vi "Session&Bearer_operation.vi"(10 "NewVal":T1(array[cluster]), 11 "OldVal":T1(array[cluster])) -> (1 "output array":T1(array[cluster]), 2 "Bearer":i32, 3 "Delete Index":i32)   [LabVIEW 2021]
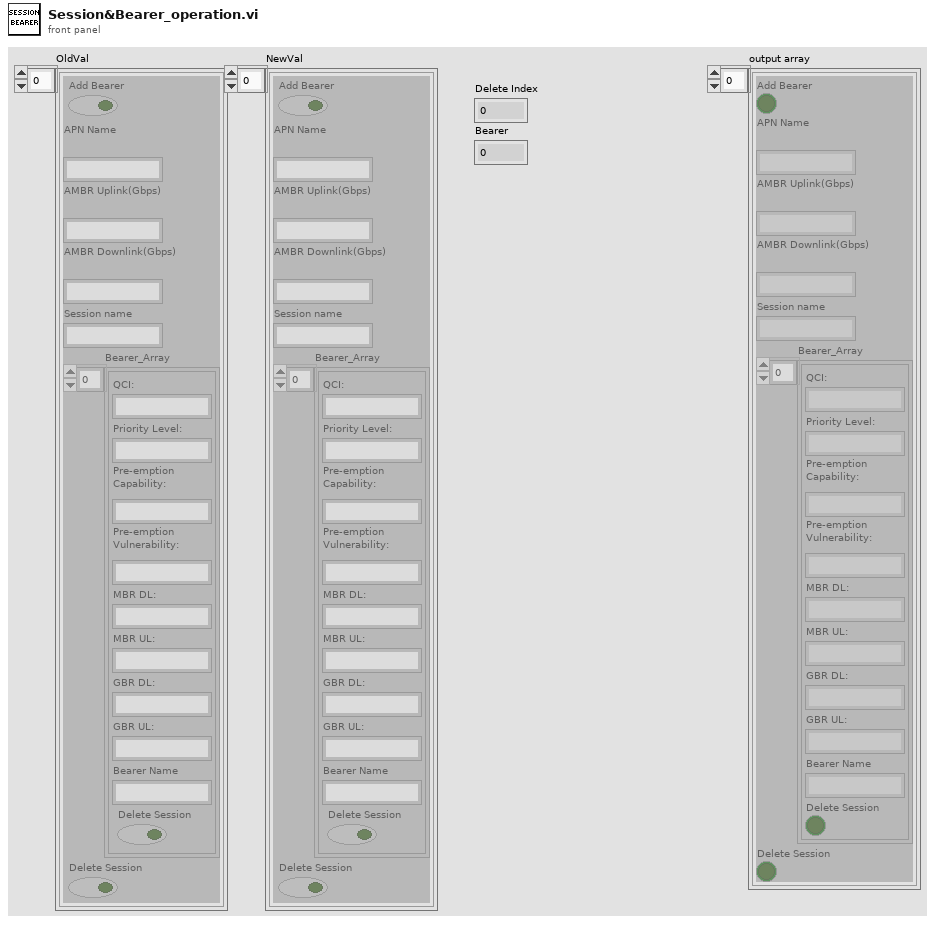
[diagram p1: front panel]
types:
  T1 = cluster{"Add Bearer":bool, "APN Name\n":string, "AMBR Uplink(Gbps)\n":string, "AMBR Downlink(Gbps)\n":string, "Session name":string, "Bearer_Array":cluster{"QCI:":string, "Priority Level:":string, "Pre-emption\nCapability:":string, "Pre-emption\nVulnerability:":string, "MBR DL:":string, "MBR UL:":string, "GBR DL:":string, "GBR UL:":string, "Bearer Name":string, "Delete Session":bool}[], "Delete Session":bool}[]
  T2 = cluster{"Add Bearer":bool, "APN Name\n":string, "AMBR Uplink(Gbps)\n":string, "AMBR Downlink(Gbps)\n":string, "Session name":string, "Bearer_Array":cluster{"QCI:":string, "Priority Level:":string, "Pre-emption\nCapability:":string, "Pre-emption\nVulnerability:":string, "MBR DL:":string, "MBR UL:":string, "GBR DL:":string, "GBR UL:":string, "Bearer Name":string, "Delete Session":bool}[], "Delete Session":bool}
  T3 = cluster{"QCI:":string, "Priority Level:":string, "Pre-emption\nCapability:":string, "Pre-emption\nVulnerability:":string, "MBR DL:":string, "MBR UL:":string, "GBR DL:":string, "GBR UL:":string, "Bearer Name":string, "Delete Session":bool}[]
  T4 = cluster{"QCI:":string, "Priority Level:":string, "Pre-emption\nCapability:":string, "Pre-emption\nVulnerability:":string, "MBR DL:":string, "MBR UL:":string, "GBR DL:":string, "GBR UL:":string, "Bearer Name":string, "Delete Session":bool}
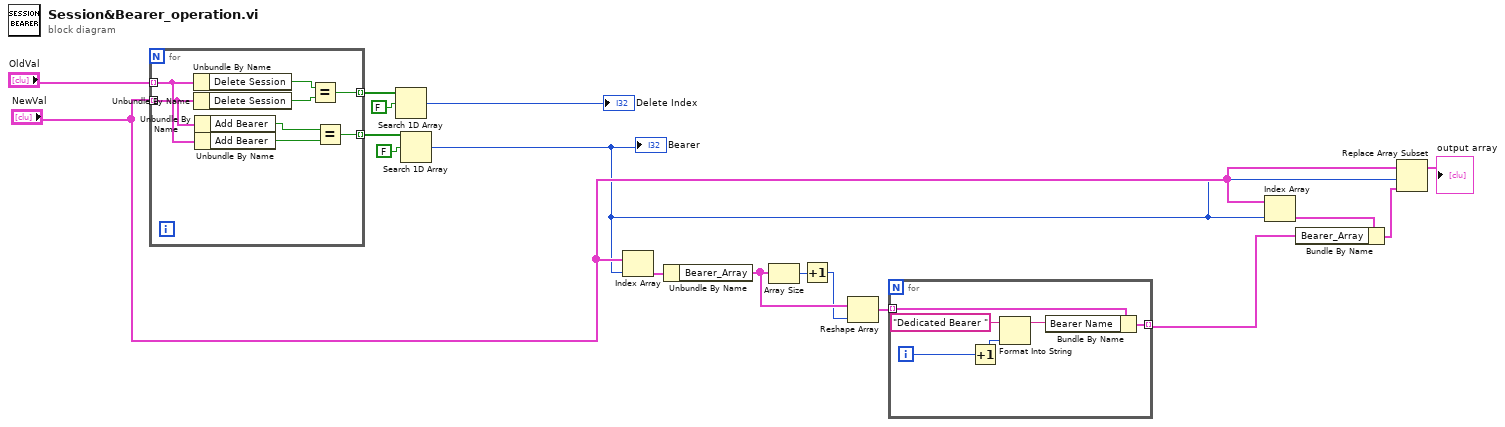
[diagram p0: block diagram]
diagram:
  n1 = for {
    tunnel: "OldVal" -> [w19] mode=indexing
    tunnel: "NewVal" -> [w18] mode=indexing
    tunnel: [w23] -> w17 mode=indexing
    tunnel: [w20] -> w13 mode=indexing
    n2 = Unbundle By Name(w19) -> ("Delete Session"=w25:bool)
    n3 = Unbundle By Name(w18) -> ("Delete Session"=w24:bool)
    n4 = Unbundle By Name(w18) -> ("Add Bearer"=w22:bool)
    n5 = Unbundle By Name(w19) -> ("Add Bearer"=w21:bool)
    n6 = Equal?(x=w25, y=w24) -> (x = y?=w23:bool)
    n7 = Equal?(x=w22, y=w21) -> (x = y?=w20:bool)
  }
  n8 = Search 1D Array(1D array=w17, element=FALSE ("x = y?")) -> (index of element=→"Delete Index":i32)  [unwired: 1 in]
  n9 = Search 1D Array(1D array=w13, element=FALSE ("x = y?")) -> (index of element=w1:i32)  [unwired: 1 in]
  "Bearer" <- w1
  n10 = Index Array(array="NewVal", index=w1) -> (element=w12:T2)
  n11 = Unbundle By Name(w12) -> ("Bearer_Array"=w11:T3)
  n12 = Array Size(array=w11) -> (size(s)=w10:i32)
  n13 = Increment(x=w10) -> (x+1=w9:i32)
  n14 = Reshape Array(w11, w9) -> (w8:T3)
  n15 = for {
    tunnel: w8 -> [w31] mode=indexing
    tunnel: [w26] -> w4 mode=indexing
    i -> [w28]
    n16 = Increment(x=w28) -> (x+1=w27:i32)
    n17 = Format Into String(initial string="Dedicated Bearer ", w27) -> (resulting string=w30:string)  [unwired: 2 in, 1 out]
    n18 = Bundle By Name(cluster=w31, "Bearer Name"=w30) -> (w26:T4)
  }
  n19 = Index Array(array="NewVal", index=w1) -> (element=w5:T2)
  n20 = Bundle By Name(cluster=w5, "Bearer_Array"=w4) -> (w3:T2)
  n21 = Replace Array Subset(array="NewVal", new element=w3, index=w1) -> (→"output array":T1)
